vi "Matrix Representation.vi"(8 "error in":errorcluster, 11 "Orient3d in":refnum<class "Orient3d Class.lvclass">) -> (0 "error out":errorcluster, 2 "Rotation Matrix":T1, 3 "Orient3d out":refnum<class "Orient3d Class.lvclass">)   [LabVIEW 2017, in "Orient3d Class.lvclass"]
uses:
  Orient3d Class.lvclass
  <vilib>/Analysis/Matrix/Datatypes/RealMatrix.ctl
  Orient3d Class.lvclass/Orient3d Class.ctl
  <vilib>/Analysis/Matrix/NI_Matrix.lvlib
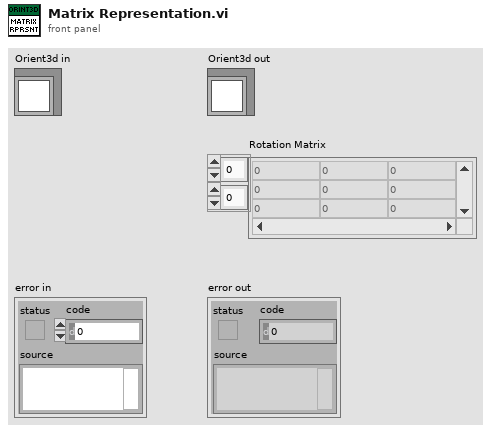
[diagram p1: front panel]
types:
  T1 = typedef "NI_Matrix.lvlib/RealMatrix.ctl" = dbl[][]
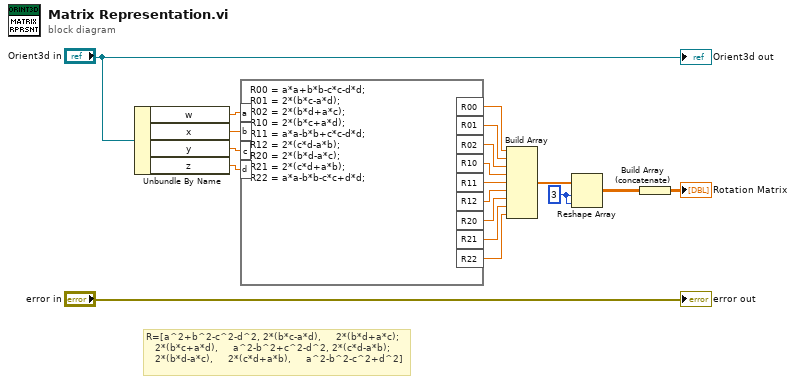
[diagram p0: block diagram]
diagram:
  w7 = 3 ("dimension size")
  # "R=[a^2+b^2-c^2-d^2, 2*(b*c-a*d),     2*(b*d+a*c);\n   2*(b*c+a*d),     a^2-b^2+c^2-d^2, 2*(c*d-a*b);\n   2*(b*d-a*c),     2*(c*d+a*b),     a^2-b^2-c^2+d^2]"
  n1 = Unbundle By Name("Orient3d in") -> ("w"=w6:dbl, "x"=w5:dbl, "y"=w4:dbl, "z"=w3:dbl)
  n2 = formula code="R00 = a*a+b*b-c*c-d*d;\nR01 = 2*(b*c-a*d);\nR02 = 2*(b*d+a*c);\nR10 = 2*(b*c+a*d);\nR11 = a*a-b*b+c*c-d*d;\nR12 = 2*(c*d-a*b);\nR20 = 2*(b*d-a*c);\nR21 = 2*(c*d+a*b);\nR22 = a*a-b*b-c*c+d*d;"("a"=w6, "b"=w5, "c"=w4, "d"=w3) -> ("R00"=w17:dbl, "R01"=w16:dbl, "R02"=w15:dbl, "R10"=w14:dbl, "R11"=w13:dbl, "R12"=w12:dbl, "R20"=w11:dbl, "R21"=w10:dbl, "R22"=w9:dbl)
  n3 = Build Array(w17, w16, w15, w14, w13, w12, w11, w10, w9) -> (w8:dbl[])
  n4 = Reshape Array(w8, w7, w7) -> (w2:dbl[][])
  n5 = Build Array (concatenate)(w2) -> (→"Rotation Matrix":T1)
  "error out" <- "error in"
  "Orient3d out" <- "Orient3d in"
